vi "Sagar C V RLC Circuit.vi"() -> ()   [LabVIEW 2018]
panel:
  in  "stop":bool
  out "XY Graph":cluster{"Y":dbl[], "Y":dbl[]}[](graph)
  out "Current":dbl
  out "Impedance":dbl
  out "Xc":dbl
  out "XL":dbl
  in  "Capacitance":dbl
  in  "Impedance":dbl
  in  "Resistance":dbl
  in  "Vin":dbl
  out "Frequency":dbl
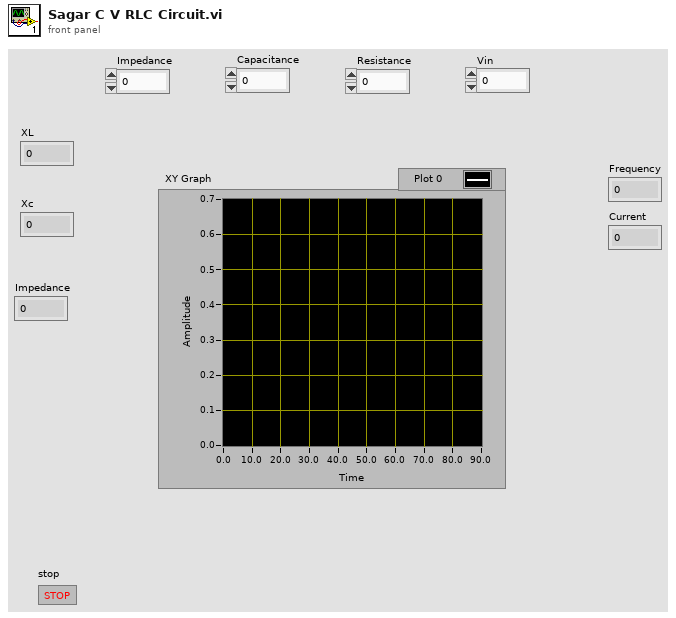
[diagram p1: front panel]
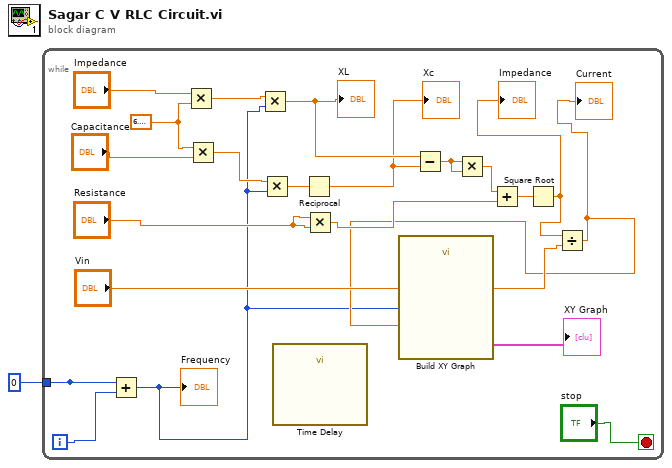
[diagram p0: block diagram]
diagram:
  n1 = while {
    tunnel: 0 -> [w21]
    tunnel: [w21] -> _
    i -> [w22]
    stop <- "stop" stop-if-true
    w20 = 6.283185307179586
    n2 = Add(x=w21, y=w22) -> (x+y=w2:i32)
    "Frequency" <- w2
    n3 = Multiply(x="Impedance", y=w20) -> (x*y=w17:dbl)
    n4 = Multiply(x=w20, y="Capacitance") -> (x*y=w16:dbl)
    n5 = Multiply(x=w17, y=w2) -> (x*y=w14:dbl)
    "XL" <- w14
    n6 = Multiply(x=w16, y=w2) -> (x*y=w15:dbl)
    n7 = call "Time Delay"() -> ()  [unwired: 11 in, 1 out]
    n8 = Reciprocal(x=w15) -> (1/x=w13:dbl)
    "Xc" <- w13
    n9 = Multiply(x="Resistance", y="Resistance") -> (x*y=w9:dbl)
    n10 = Subtract(x=w14, y=w13) -> (x-y=w12:dbl)
    n11 = Multiply(x=w12, y=w12) -> (x*y=w10:dbl)
    n12 = Add(x=w10, y=w9) -> (x+y=w8:dbl)
    n13 = Square Root(x=w8) -> (sqrt(x)=w6:dbl)
    "Impedance" <- w6
    n14 = Divide(x=w6, y="Vin") -> (x/y=w3:dbl)
    "Current" <- w3
    n15 = call "Build XY Graph"("Y Input"=w3, "X Input"=w2) -> ("XY Graph"=→"XY Graph":cluster{"X":dbl[], "Y":dbl[]}[])  [unwired: 8 in, 1 out]
  }
